vi "dfd_Check Frequency Vector.vi"(6 "fs [Hz] in":dbl=-1.0 format="%.2f", 7 "frequency vector":dbl[](array[numeric]), 8 "error in (no error)":errorcluster, 10 "filter fs[Hz]":dbl) -> (0 "error out":errorcluster, 4 "fs out [Hz]":dbl, 5 "frequency vector out":dbl[](array[numeric]))   [LabVIEW 2017, in "NI_DigFilterLicensed.lvlib"]
uses:
  <vilib>/addons/Digital Filter Design/NI_DigFilterLicensed.lvlib
  <vilib>/addons/Digital Filter Design/_Misc.llb/dfd_Error Handlers (Single).vi
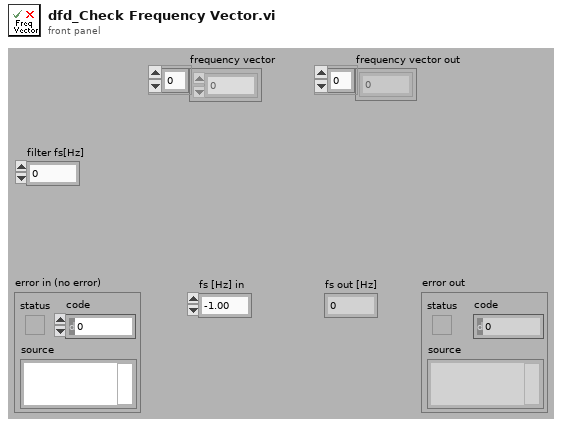
[diagram p1: front panel]
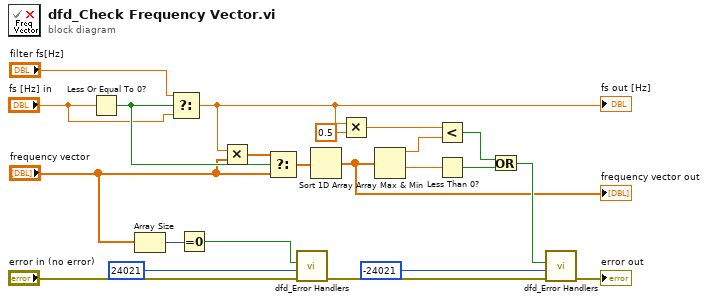
[diagram p0: block diagram]
diagram:
  n1 = Less Or Equal To 0?(x="fs [Hz] in") -> (x <= 0?=w17:bool)
  n2 = Array Size(array="frequency vector") -> (size(s)=w5:i32)
  n3 = Select(t="filter fs[Hz]", s=w17, f="fs [Hz] in") -> (s? t:f=w12:dbl)
  "fs out [Hz]" <- w12
  n4 = Equal To 0?(x=w5) -> (x = 0?=w1:bool)
  n5 = Multiply(x=w12, y="frequency vector") -> (x*y=w13:dbl[])
  n6 = Select(t=w13, s=w17, f="frequency vector") -> (s? t:f=w16:dbl[])
  n7 = call-poly <vilib>:"dfd_Error Handlers.vi"("error in (no error)"="error in (no error)", "error code"=24021 ("WRN_EMPTY_FREQ_VECTOR"), "condition failed?"=w1) -> ("error out"=w2:errorcluster)  [unwired: 8 out]
  n8 = Sort 1D Array(array=w16) -> (sorted array=w7:dbl[])
  "frequency vector out" <- w7
  n9 = Multiply(x=w12, y=0.5) -> (x*y=w19:dbl)
  n10 = Array Max & Min(array=w7) -> (max value=w10:dbl, min value=w11:dbl)  [unwired: 2 out]
  n11 = Less?(x=w19, y=w10) -> (x < y?=w9:bool)
  n12 = Less Than 0?(x=w11) -> (x < 0?=w8:bool)
  n13 = Or(x=w9, y=w8) -> (x .or. y?=w18:bool)
  n14 = call-poly <vilib>:"dfd_Error Handlers.vi"("error in (no error)"=w2, "error code"=-24021 ("ERR_FREQ_RANGE_WRONG"), "condition failed?"=w18) -> ("error out"=→"error out":errorcluster)  [unwired: 8 out]
